vi "var_num_v3.vi"() -> ()   [LabVIEW 2009]
panel:
  out "Afisare grafica valoare numerica":i32(graph)
  in  "Introducere valoare numerica":i32(knob) scale=0.0..100.0
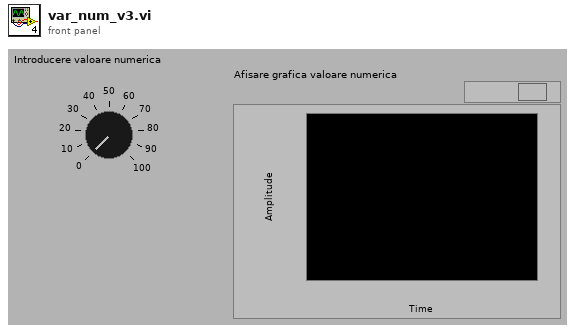
[diagram p1: front panel]
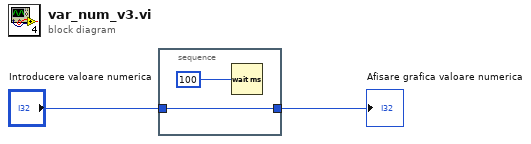
[diagram p0: block diagram]
diagram:
  n1 = stacked-sequence {
    tunnel: "Introducere valoare numerica" -> [w3]
    tunnel: [w3] -> w1
    frame #0 {
      n2 = Wait (ms)(milliseconds to wait=100) -> ()  [unwired: 1 out]
    }
  }
  "Afisare grafica valoare numerica" <- w1
